vi "Read State.vi"(8 "error in (no error)":errorcluster, 11 "B State in":refnum<class "B State.lvclass">) -> (0 "error out":errorcluster, 2 "State":refnum<class "State Pattern.lvclass">, 3 "B State out":refnum<class "B State.lvclass">)   [LabVIEW 2021, in "Context.lvlib" / "B State.lvclass"]
uses:
  B State.lvclass
  B State.lvclass/B State.ctl
  Context/Context.lvclass
  C:/Program Files/National Instruments/LabVIEW 2021/vi.lib/ActorFramework/Actor/Actor.lvclass
  C:/PPLs/Design-Patterns/State Pattern/State Pattern/State Change Core/State Change Core/State Change Core.lvclass
  C:/PPLs/Design-Patterns/State Pattern/State Pattern/State Pattern/State Pattern.lvclass
  C:/PPLs/Design-Patterns/State Pattern/Example/Context/State/State.lvclass
  C:/PPLs/Design-Patterns/State Pattern/Example/Context/Context/Context.lvclass
  C:/PPLs/Design-Patterns/State Pattern/Example/Messages/Flip States/Flip States/Flip States.lvclass
  C:/PPLs/Design-Patterns/State Pattern/Example/Messages/xxxx/xxxx/xxxx.lvclass
  State Pattern/State Pattern/State Pattern.lvclass
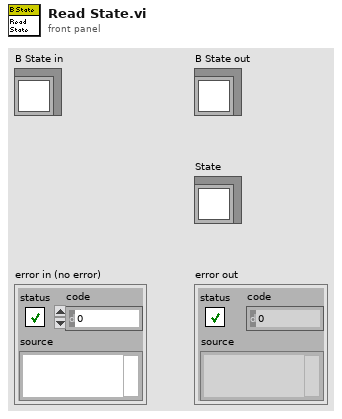
[diagram p1: front panel]
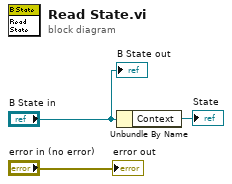
[diagram p0: block diagram]
diagram:
  n1 = Unbundle By Name("B State in") -> ("Context"=→"State":refnum<class "Context.lvclass">)
  "error out" <- "error in (no error)"
  "B State out" <- "B State in"
